vi "Test Data Dictionary API.vi"(8 "error in (no error)":errorcluster) -> (0 "error out":errorcluster)   [LabVIEW 2016]
uses:
  Data/Typedefs/Dictionary--cluster.ctl
  Data/Data.lvclass
  Data/Data.lvclass/Data.ctl
  <vilib>/addons/_JKI Toolkits/Caraya/classes/Assert/Assert Not Error.vi
  <vilib>/addons/_JKI Toolkits/Caraya/classes/Assert/Assert Equal Value and Type_Variant.vi
  Data/Protected/Variant to Array.vi
  <vilib>/addons/_JKI Toolkits/Caraya/classes/Assert/Assert True.vi
  <vilib>/addons/_JKI Toolkits/Caraya/classes/Assert/Assert.lvclass
  <vilib>/addons/_JKI Toolkits/Caraya/classes/Test/Test.lvclass
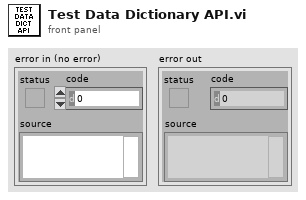
[diagram p1: front panel]
types:
  T1 = typedef "Data.lvclass/Dictionary--cluster.ctl" = cluster{"key":string, "value":variant}
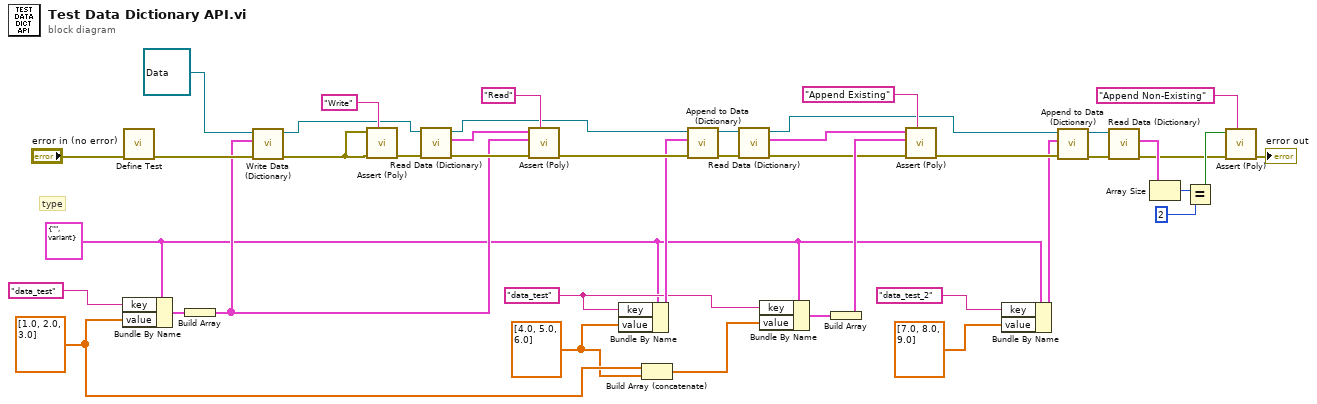
[diagram p0: block diagram]
diagram:
  w24 = "data_test" ("key")
  w2 = dbl[] [4.0, 5.0, 6.0]
  w12 = T1 {"key"="", "value"=variant} ("key-value")
  w3 = dbl[] [1.0, 2.0, 3.0]
  # "type"
  n1 = Bundle By Name(cluster=w12, "key"="data_test", "value"=w3) -> (w41:T1)
  n2 = call <vilib>:"Define Test.vi"("error in (no error)"="error in (no error)") -> ("error out"=w40:errorcluster)  [unwired: 10 in]
  n3 = Build Array(w41) -> (w33:T1[])
  n4 = call "Write Data (Dictionary).vi"("error in (no error)"=w40, "Data (Dictionary)"=w33, "Data Save"=refnum<class "Data.lvclass"> refnum) -> ("error out"=w37:errorcluster, "Data Save out"=w32:refnum<class "Data.lvclass">)  [unwired: 7 in]
  n5 = call-poly <vilib>:"Assert (Poly).vi"("Label"="Write", "error in (no error)"=w37, "Not Error?"=w37) -> ("error out"=w38:errorcluster)  [unwired: 8 in]
  n6 = call "Read Data (Dictionary).vi"("error in (no error)"=w38, "Data Save"=w32) -> ("error out"=w36:errorcluster, "Data (Dictionary)"=w34:T1[], "Data Save out"=w29:refnum<class "Data.lvclass">)  [unwired: 7 in]
  n7 = call-poly <vilib>:"Assert (Poly).vi"("Label"="Read", "error in (no error)"=w36, "Y"=w33, "X"=w34) -> ("error out"=w30:errorcluster)  [unwired: 7 in]
  n8 = Bundle By Name(cluster=w12, "key"=w24, "value"=w2) -> (w28:T1)
  n9 = Build Array (concatenate)(w3, w2) -> (w25:dbl[])
  n10 = call "Append to Data (Dictionary).vi"("error in (no error)"=w30, "key-value"=w28, "Data Save"=w29) -> ("error out"=w27:errorcluster, "Data Save out"=w26:refnum<class "Data.lvclass">)  [unwired: 7 in]
  n11 = call "Read Data (Dictionary).vi"("error in (no error)"=w27, "Data Save"=w26) -> ("error out"=w20:errorcluster, "Data (Dictionary)"=w21:T1[], "Data Save out"=w15:refnum<class "Data.lvclass">)  [unwired: 7 in]
  n12 = Bundle By Name(cluster=w12, "key"=w24, "value"=w25) -> (w23:T1)
  n13 = Build Array(w23) -> (w22:T1[])
  n14 = call-poly <vilib>:"Assert (Poly).vi"("Label"="Append Existing", "error in (no error)"=w20, "Y"=w22, "X"=w21) -> ("error out"=w16:errorcluster)  [unwired: 7 in]
  n15 = Bundle By Name(cluster=w12, "key"="data_test_2", "value"=dbl[] [7.0, 8.0, 9.0]) -> (w11:T1)
  n16 = call "Append to Data (Dictionary).vi"("error in (no error)"=w16, "key-value"=w11, "Data Save"=w15) -> ("error out"=w17:errorcluster, "Data Save out"=w18:refnum<class "Data.lvclass">)  [unwired: 7 in]
  n17 = call "Read Data (Dictionary).vi"("error in (no error)"=w17, "Data Save"=w18) -> ("error out"=w6:errorcluster, "Data (Dictionary)"=w10:T1[])  [unwired: 7 in, 1 out]
  n18 = Array Size(array=w10) -> (size(s)=w9:i32)
  n19 = Equal?(x=w9, y=2) -> (x = y?=w7:bool)
  n20 = call-poly <vilib>:"Assert (Poly).vi"("Label"="Append Non-Existing", "error in (no error)"=w6, "True?"=w7) -> ("error out"=→"error out":errorcluster)  [unwired: 8 in]
